vi "Processing Step.vi"(8 "error in (no error)":errorcluster, 11 "SSE Handler in":refnum<class "SSE Handler.lvclass">) -> (0 "error out":errorcluster, 2 "Step":T1[](array[typedef]), 3 "SSE Handler out":refnum<class "SSE Handler.lvclass">)   [LabVIEW 2020, in "HTTP Server.lvlib" / "SSE Handler.lvclass"]
uses:
  SSE Handler.lvclass
  Processing Step.ctl
  SSE Handler.lvclass/SSE Handler.ctl
  HTTP Server.lvlib
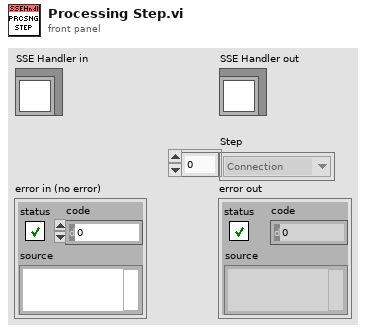
[diagram p1: front panel]
types:
  T1 = typedef "HTTP Server.lvlib/Processing Step.ctl" = enum16{"Connection", "Request", "Routing", "Controller Init", "Controller", "Response", "Complete", "Exception"}
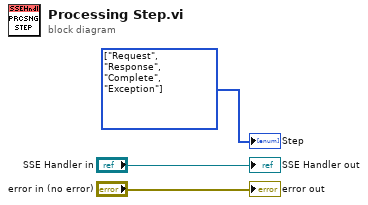
[diagram p0: block diagram]
diagram:
  w1 = T1[] [enum."Request", enum."Response", enum."Complete", enum."Exception"] items=["Connection", "Request", "Routing", "Controller Init", "Controller", "Response", "Complete", "Exception"] ("Array")
  "error out" <- "error in (no error)"
  "SSE Handler out" <- "SSE Handler in"
  "Step" <- w1
